vi "acquisitionGetVolume.vi"(4 "volumeDirectionReferences":refnum<data-value>[](array[refnum]), 6 "hamamatsuFrameAvailableReferences":refnum<data-value>[](array[refnum]), 7 "volumeFirstFrameReferences":refnum<data-value>[](array[refnum]), 8 "hamamatsuFrameReferences":refnum<data-value>[](array[refnum]), 9 "volume index (last: 1)":i32=1) -> (0 "success":bool, 1 "numberOfFrames":u32, 2 "absoluteCountFirstFrame":u32, 3 "volume out":u16[][][](array[numeric]), 5 "volume direction out":bool)   [LabVIEW 2017]
uses:
  globalUtilities.vi
  globalDevices.vi
panel:
  # "0th is the one which just had its\nfirstFrame, but not the last one."
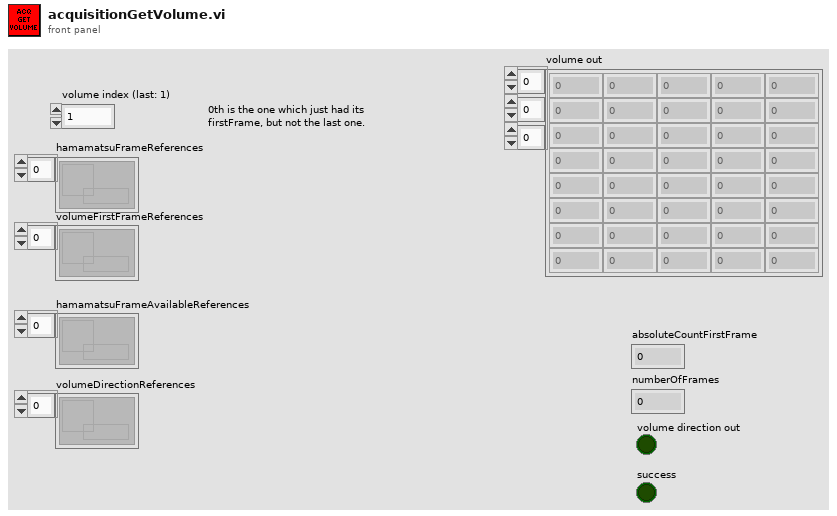
[diagram p1: front panel]
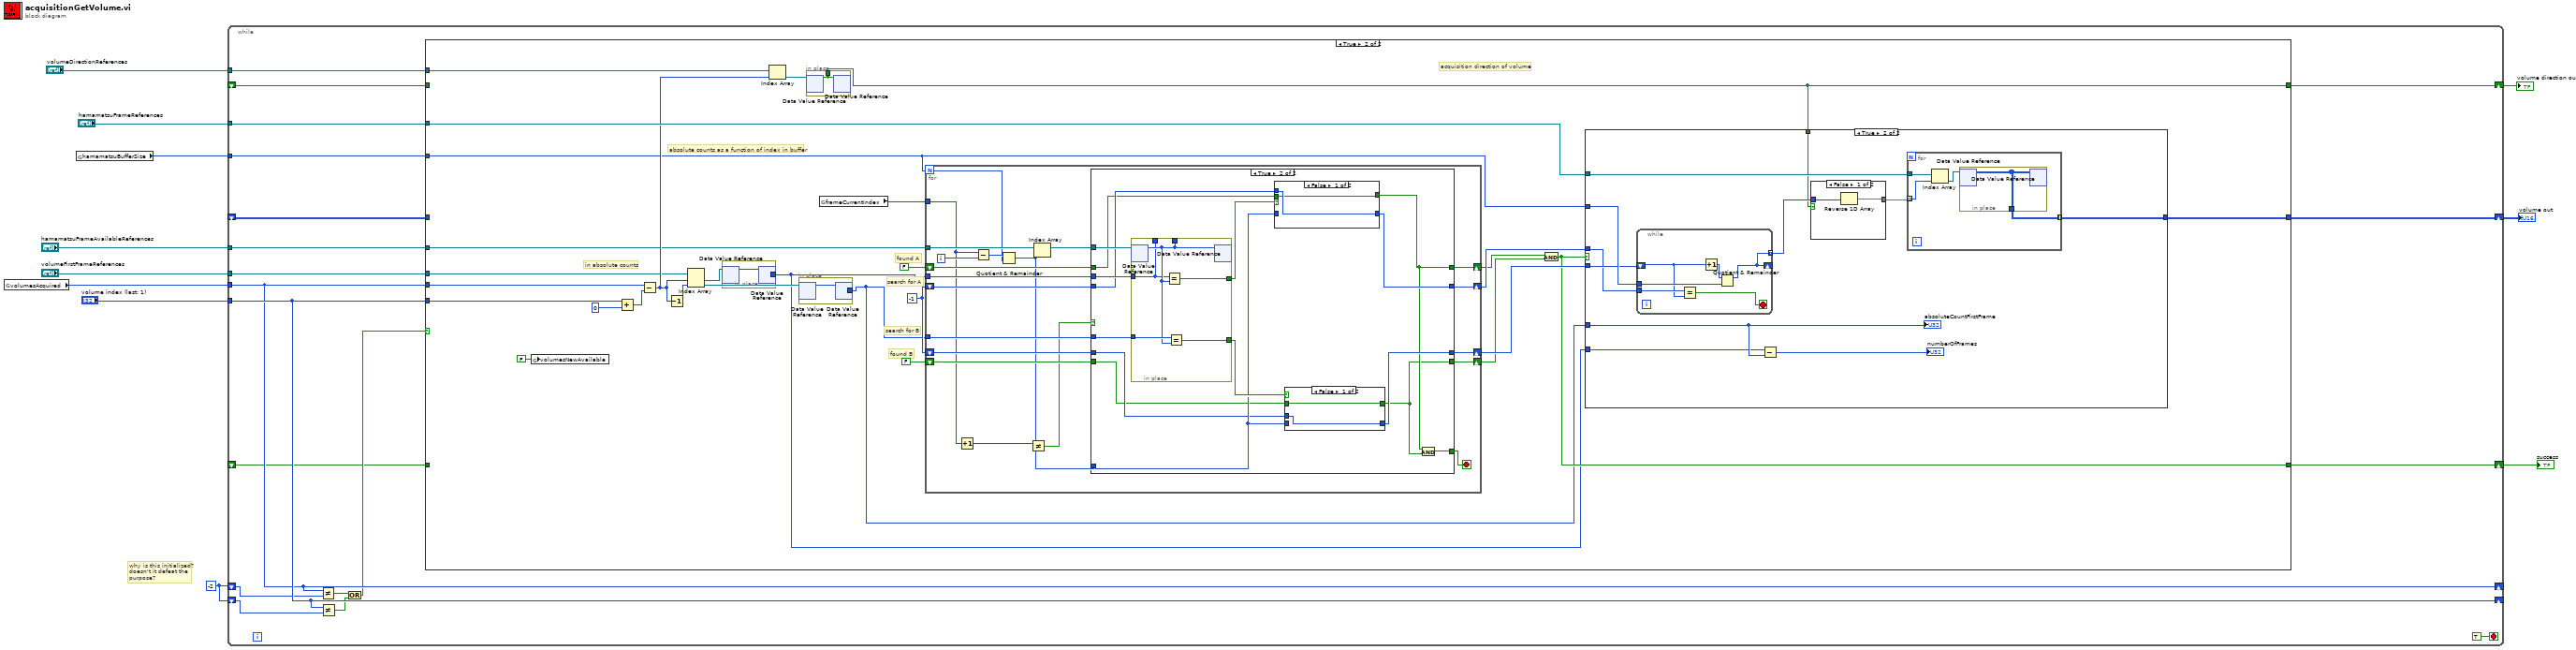
[diagram p0: block diagram]
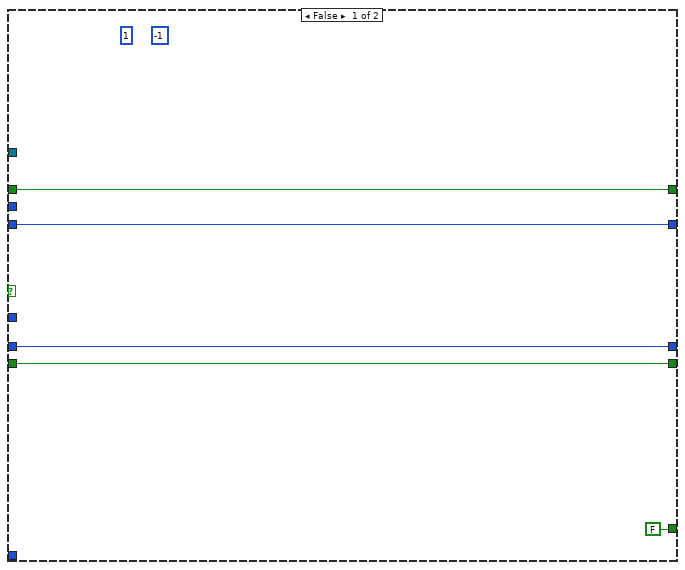
[diagram p3: hidden frame]
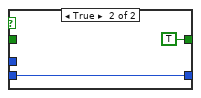
[diagram p4: hidden frame]
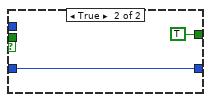
[diagram p5: hidden frame]
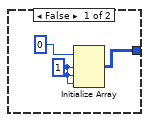
[diagram p6: hidden frame]
diagram:
  w1 = -2 ("volumesAcquired")
  # "why is this initialized?\ndoesn't it defeat the\npurpose?"
  n1 = global read "globalUtilities.vi" "volumesAcquired"() -> (w8:i32)
  n2 = global read "globalDevices.vi" "hamamatsuBufferSize"() -> (w6:i32)
  n3 = while {
    tunnel: "hamamatsuFrameReferences" -> [w30]
    tunnel: "hamamatsuFrameAvailableReferences" -> [w29]
    tunnel: "volumeDirectionReferences" -> [w28]
    tunnel: w8 -> [w19]
    tunnel: "volumeFirstFrameReferences" -> [w27]
    tunnel: w6 -> [w26]
    shift-right: [w25] -> w5
    shift-left: _ -> [w14]
    shift-right: [w23] -> w3
    shift-left: _ -> [w15]
    shift-right: [w24] -> w4
    shift-left: _ -> [w13]
    shift-right: [w22] -> _
    shift-left: w1 -> [w21]
    shift-right: [w19] -> _
    shift-left: w1 -> [w20]
    tunnel: "volume index (last: 1)" -> [w22]
    stop <- TRUE stop-if-true
    n4 = Not Equal?(x=w19, y=w20) -> (x != y?=w18:bool)
    n5 = Not Equal?(x=w22, y=w21) -> (x != y?=w17:bool)
    n6 = Or(x=w18, y=w17) -> (x .or. y?=w16:bool)
    n7 = case shown="True" w16 {
      tunnel: w22 -> [_ w58]
      tunnel: w30 -> [_ w57]
      tunnel: w29 -> [_ w55]
      tunnel: w28 -> [_ w52]
      tunnel: w19 -> [_ w50]
      tunnel: w27 -> [_ w49]
      tunnel: w26 -> [_ w43]
      tunnel: [w33 w39] -> w25
      tunnel: [w31 w38] -> w24
      tunnel: [w32 w37] -> w23
      tunnel: w15 -> [w32 _]
      tunnel: w14 -> [w33 _]
      tunnel: w13 -> [w31 _]
      frame False {
      }
      frame True {
        w45 = -1 ("f")
        # "search for B"
        # "found B"
        # "search for A"
        # "found A"
        # "acquisition direction of volume"
        # "absolute counts as a function of index in buffer"
        # "in absolute counts"
        n8 = global write "globalUtilities.vi" "volumesNewAvailable"(FALSE) -> ()
        n9 = Add(x=w58, y=0) -> (x+y=w60:i32)
        n10 = Subtract(x=w50, y=w60) -> (x-y=w56:i32)
        n11 = Decrement(x=w56) -> (x-1=w61:i32)
        n12 = Index Array(array=w49, index #1=w56, index #2=w61) -> (element #1=w48:refnum<data-value>, element #2=w47:refnum<data-value>)
        n13 = in-place {
          in-place-border: [w63] -> w36
          n14 = in-place-dvr #1(w48) -> (w63:u32)  [unwired: 1 out]
          n15 = in-place-dvr #1(w63) -> ()  [unwired: 2 out]
        }
        n16 = Index Array(array=w52, index=w56) -> (element=w51:refnum<data-value>)
        n17 = in-place {
          in-place-border: [w62] -> w35
          n18 = in-place-dvr #2(w47) -> (w62:u32)  [unwired: 1 out]
          n19 = in-place-dvr #2(w62) -> ()  [unwired: 2 out]
        }
        n20 = in-place {
          in-place-border: [w64] -> w37
          n21 = in-place-dvr #3(w51) -> (w64:bool)  [unwired: 1 out]
          n22 = in-place-dvr #3(w64) -> ()  [unwired: 2 out]
        }
        n23 = global read "globalUtilities.vi" "frameCurrentIndex"() -> (w42:i32)
        n24 = for {
          N: w43 -> [w68]
          tunnel: w55 -> [w83]
          shift-right: [w74] -> w41
          shift-left: FALSE -> [w78]
          tunnel: w36 -> [w82]
          shift-right: [w80] -> w53
          shift-left: w45 -> [w79]
          tunnel: w35 -> [w81]
          shift-right: [w77] -> w44
          shift-left: w45 -> [w76]
          shift-right: [w73] -> w40
          shift-left: FALSE -> [w75]
          tunnel: w42 -> [w67]
          i -> [w70]
          stop <- w66 stop-if-true
          n25 = Increment(x=w67) -> (x+1=w84:i32)
          n26 = Subtract(x=w67, y=w70) -> (x-y=w69:i32)
          n27 = Quotient & Remainder(x=w69, y=w68) -> (x-y*floor(x/y)=w65:i32)  [unwired: 1 out]
          n28 = Not Equal?(x=w84, y=w65) -> (x != y?=w72:bool)
          n29 = Index Array(array=w83, index=w65) -> (element=w71:refnum<data-value>)
          n30 = case shown="True" w72 {
            tunnel: w71 -> [_ w104]
            tunnel: w82 -> [_ w103]
            tunnel: w81 -> [_ w102]
            tunnel: [w88 w100] -> w80
            tunnel: w79 -> [w88 w99]
            tunnel: w78 -> [w89 w98]
            tunnel: w65 -> [_ w96]
            tunnel: [w87 w95] -> w77
            tunnel: w76 -> [w87 w94]
            tunnel: w75 -> [w86 w93]
            tunnel: [FALSE w92] -> w66
            tunnel: [w89 w91] -> w74
            tunnel: [w86 w90] -> w73
            frame False {
              (unwired) u32 1 ("element")
              (unwired) -1
            }
            frame True {
              n31 = in-place {
                in-place-border: w103 -> [w113]
                in-place-border: [w117] -> w101
                in-place-border: w102 -> [w116]
                in-place-border: [w115] -> w97
                in-place-border: [w114] -> _
                in-place-border: [w113] -> _
                n32 = in-place-dvr #4(w104) -> (w114:i32)  [unwired: 1 out]
                n33 = Equal?(x=w113, y=w114) -> (x = y?=w117:bool)
                n34 = Equal?(x=w116, y=w114) -> (x = y?=w115:bool)
                n35 = in-place-dvr #4(w114) -> ()  [unwired: 2 out]
              }
              n36 = case shown="False" w101 {
                tunnel: w96 -> [_ w112]
                tunnel: [w110 w112] -> w100
                tunnel: w99 -> [w110 _]
                tunnel: w98 -> [w109 _]
                tunnel: [w109 TRUE] -> w91
                frame False {
                }
                frame True {
                }
              }
              n37 = case shown="False" w97 {
                tunnel: w96 -> [_ w108]
                tunnel: [w106 w108] -> w95
                tunnel: [w105 TRUE] -> w90
                tunnel: w94 -> [w106 _]
                tunnel: w93 -> [w105 _]
                frame False {
                }
                frame True {
                }
              }
              n38 = And(x=w91, y=w90) -> (x .and. y?=w92:bool)
            }
          }
        }
        n39 = And(x=w41, y=w40) -> (x .and. y?=w38:bool)
        n40 = case shown="True" w38 {
          tunnel: w43 -> [_ w131]
          tunnel: w44 -> [_ w130]
          tunnel: w35 -> [_ w128]
          tunnel: w36 -> [_ w127]
          tunnel: w53 -> [_ w126]
          tunnel: w57 -> [_ w125]
          tunnel: w37 -> [_ w122]
          tunnel: [w118 w121] -> w39
          frame False {
            w119 = 1 ("dimension size")
            n41 = Initialize Array(u16 0, w119, w119, w119) -> (w118:u16[][][])
          }
          frame True {
            n42 = while {
              shift-right: [w140] -> _
              shift-left: w130 -> [w141]
              tunnel: w131 -> [w145]
              tunnel: w126 -> [w143]
              tunnel: [w140] -> w124 mode=indexing
              stop <- w142 stop-if-true
              n43 = Equal?(x=w143, y=w141) -> (x = y?=w142:bool)
              n44 = Increment(x=w141) -> (x+1=w144:i32)
              n45 = Quotient & Remainder(x=w144, y=w145) -> (x-y*floor(x/y)=w140:i32)  [unwired: 1 out]
            }
            n46 = Subtract(x=w127, y=w128) -> (x-y=→"numberOfFrames":u32)
            n47 = case shown="False" w122 {
              tunnel: w124 -> [w133 w134]
              tunnel: [w132 w134] -> w123
              frame False {
                n48 = Reverse 1D Array(array=w133) -> (reversed array=w132:i32[])
              }
              frame True {
              }
            }
            n49 = for {
              tunnel: w123 -> [w137] mode=indexing
              tunnel: w125 -> [w138]
              tunnel: [w135] -> w121 mode=indexing
              n50 = Index Array(array=w138, index=w137) -> (element=w136:refnum<data-value>)
              n51 = in-place {
                in-place-border: [w139] -> w135
                n52 = in-place-dvr #5(w136) -> (w139:u16[][])  [unwired: 1 out]
                n53 = in-place-dvr #5(w139) -> ()  [unwired: 2 out]
              }
            }
            "absoluteCountFirstFrame" <- w128
          }
        }
      }
    }
  }
  "volume out" <- w5
  "success" <- w4
  "volume direction out" <- w3
